vi "Pneumatic Sucker Suck.vi"(8 "error in":errorcluster, 10 "suck sec":dbl=0.8 format="%#_13g") -> (0 "error out":errorcluster)   [LabVIEW 2019]
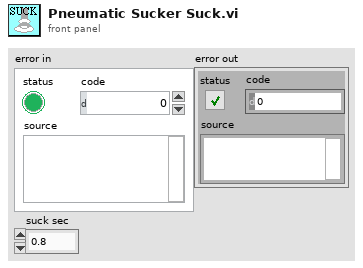
[diagram p1: front panel]
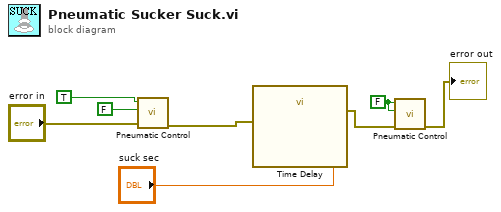
[diagram p0: block diagram]
diagram:
  w3 = FALSE ("ENA")
  n1 = call "Pneumatic Control.vi"("error in"="error in", "DIR"=FALSE, "ENA"=TRUE) -> ("error out"=w6:errorcluster)  [unwired: 8 in]
  n2 = call "Time Delay"("error in (no error)"=w6, "Delay Time (s)"="suck sec") -> ("error out"=w4:errorcluster)  [unwired: 9 in]
  n3 = call "Pneumatic Control.vi"("error in"=w4, "DIR"=w3, "ENA"=w3) -> ("error out"=→"error out":errorcluster)  [unwired: 8 in]
